vi "Process.vi"(8 "error in (no error)":errorcluster, 11 "SMO.UI.Example":refnum<class "SMO.UI.Example.lvclass">) -> (0 "error out":errorcluster, 3 "SMO.UI.Example out":refnum<class "SMO.UI.Example.lvclass">)   [LabVIEW 2013, in "SMO.UI.Example.lvclass"]
uses:
  SMO.UI.Example.lvclass
  SMO/Typedefs/Parent Call--Enum.ctl
  SMO.UI.Example.lvclass/SMO.UI.Example.ctl
  SMO.UI/SMO.UI.lvclass
  <vilib>/Utility/miscctls.llb/LVPointTypeDef.ctl
  SMO/Protected/ListThisLevelDependencies.vi
  SMO/reuse/CastArrayDependenciesToClusterOrClass.vi
  SMO.Example/SMO.Example.lvclass
  SMO/SMO.lvclass
panel:
  in  "------------ User Events -------":bool=TRUE
  out "Waveform Chart":cluster{"Flow 2":dbl, "Flow 1":dbl}(graph)
  out "Sensor 1 (LPM)":u8
  out "Sensor 2 (LPM)":u8
  in  "Valve":bool
  in  "Pump":bool
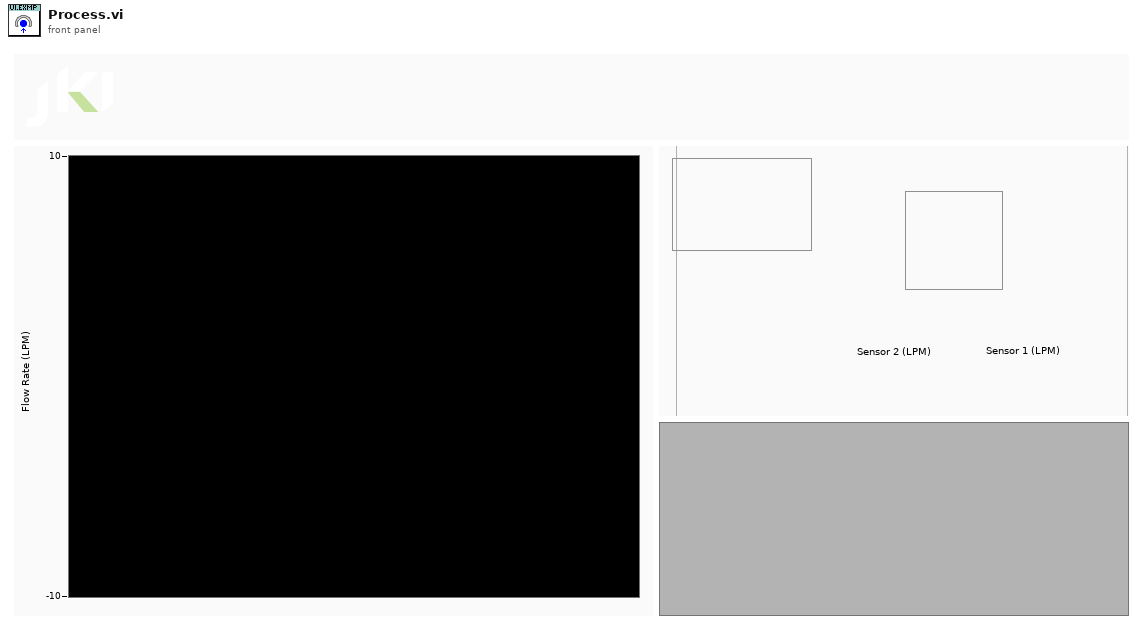
[diagram p1: front panel]
types:
  T1 = typedef "SMO.lvclass/Parent Call--Enum.ctl" = enum16{"Allows parent to run", "Does not request parent to run"}
  T2 = enum32{"invalid app kind", "Development System", "Run Time System", "Student Edition", "Embedded LabVIEW", "Evaluation", "Custom"}
  T3 = typedef "LVPointTypeDef.ctl" = cluster{"Horizontal":i16, "Vertical":i16}
  T4 = enum32{"Invalid", "Standard", "Closed", "Hidden", "Minimized", "Maximized"}
  T5 = typedef "SMO.UI.Example.lvclass/Dependencies--Cluster.ctl" = cluster{"SMO.Example":refnum<class "SMO.Example.lvclass">}
  T6 = cluster{"Core":cluster{"Current VI Reference":refnum<vi>, "Close Panel on Exit?":bool, "error":errorcluster}, "Self Ref":refnum<class "SMO.UI.Example.lvclass">, "Dependencies":T5, "Flow 1":dbl, "Flow 2":dbl}
  T7 = cluster{"Current VI Reference":refnum<vi>, "Close Panel on Exit?":bool, "error":errorcluster}
  T8 = typedef "SMO.lvclass/Protected Events.ctl" = cluster{"StopProcesses":refnum<user-event>, "AbortProcesses":refnum<user-event>, "Config Changed":refnum<user-event>}
  T9 = cluster{"Event Registration Refnum":refnum<event-registration>, "SMO.Example Public Events":refnum<event-registration>}
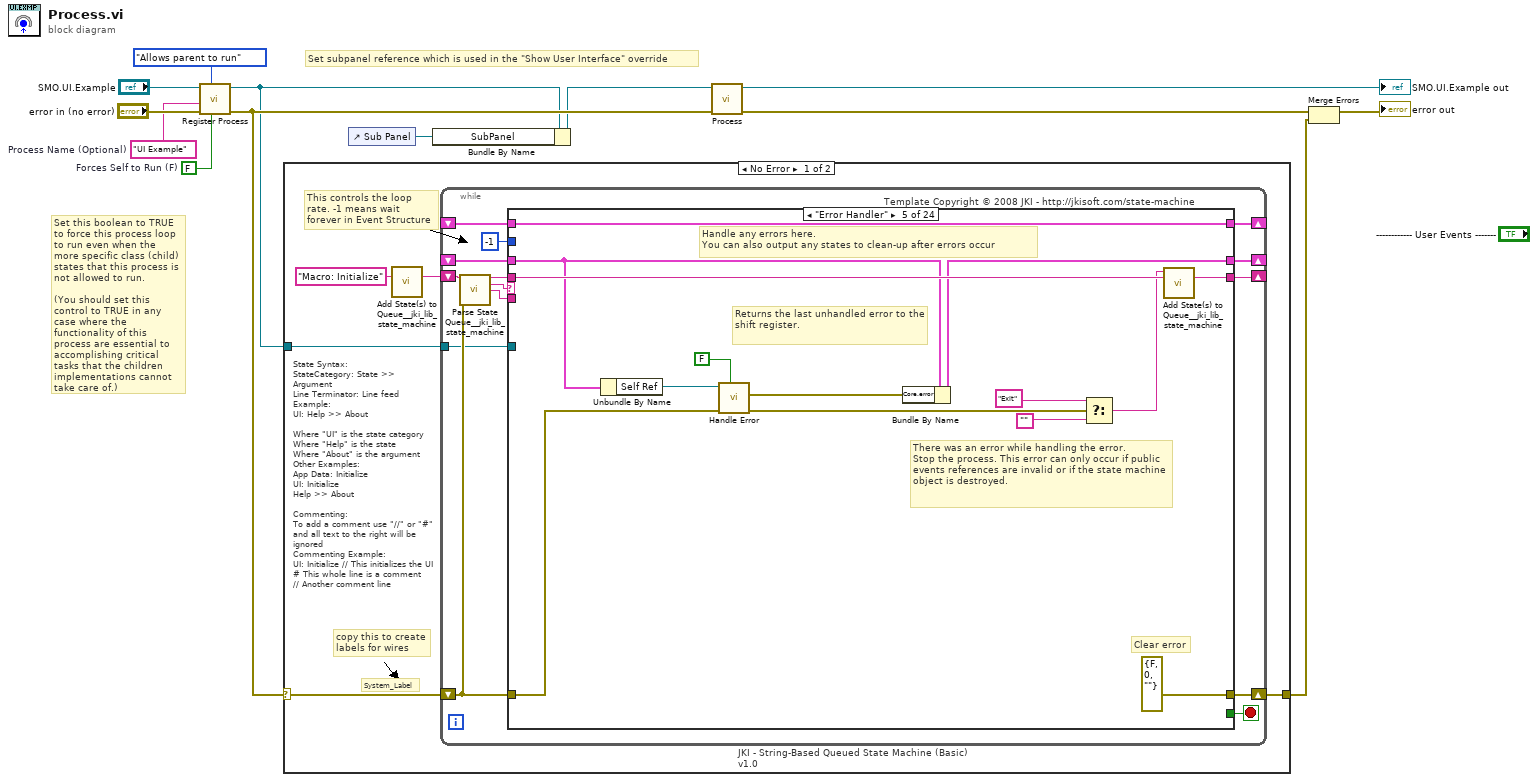
[diagram p0: block diagram]
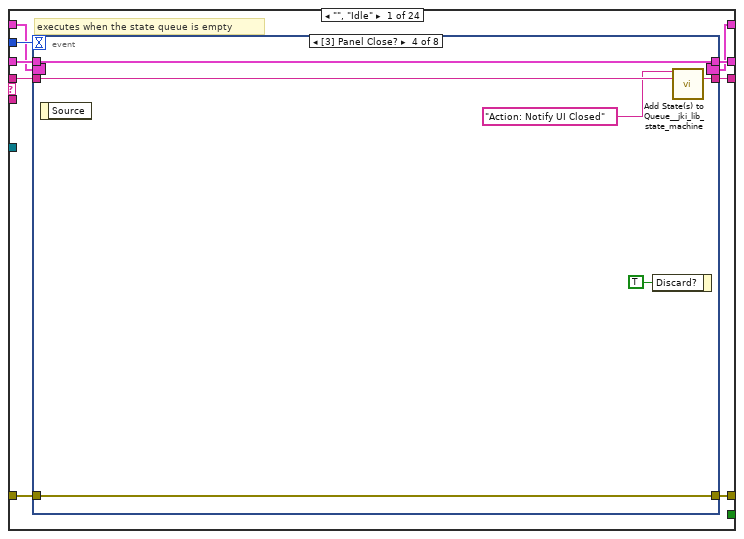
[diagram p2: hidden frame]
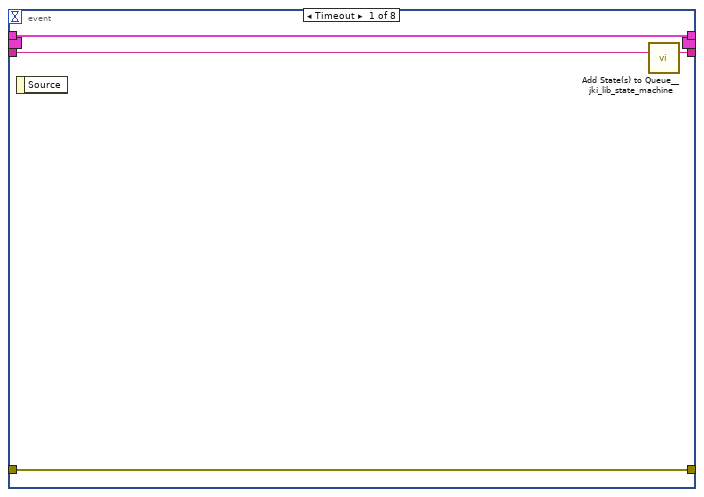
[diagram p3: hidden frame]
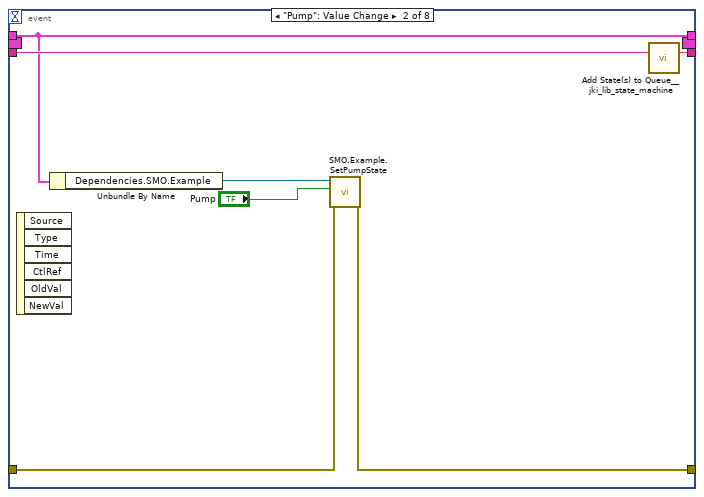
[diagram p4: hidden frame]
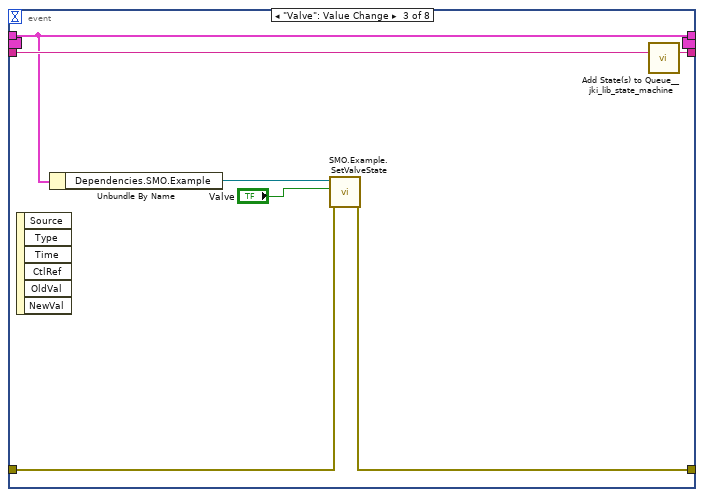
[diagram p5: hidden frame]
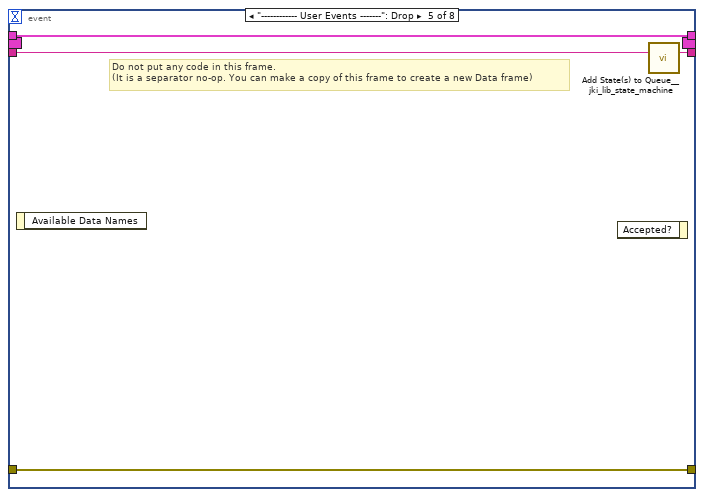
[diagram p6: hidden frame]
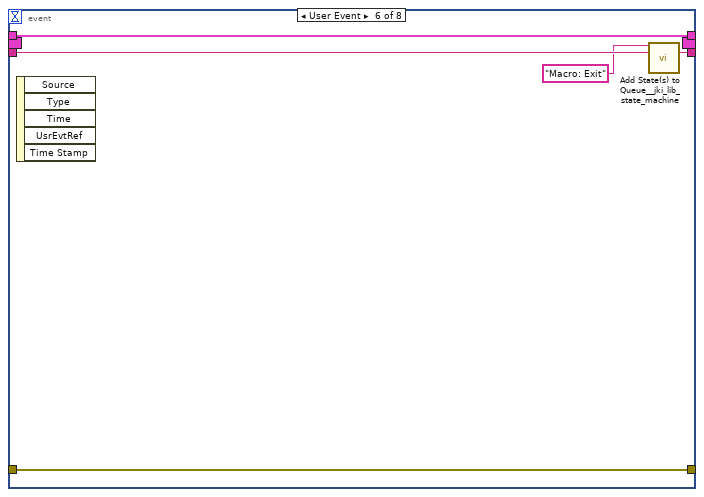
[diagram p7: hidden frame]
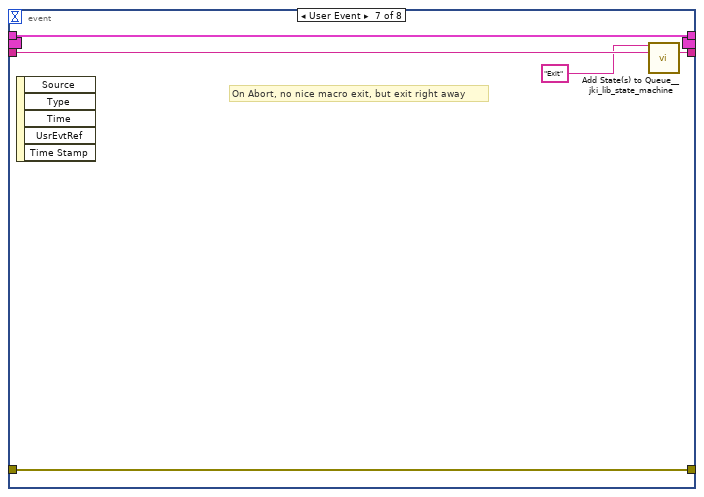
[diagram p8: hidden frame]
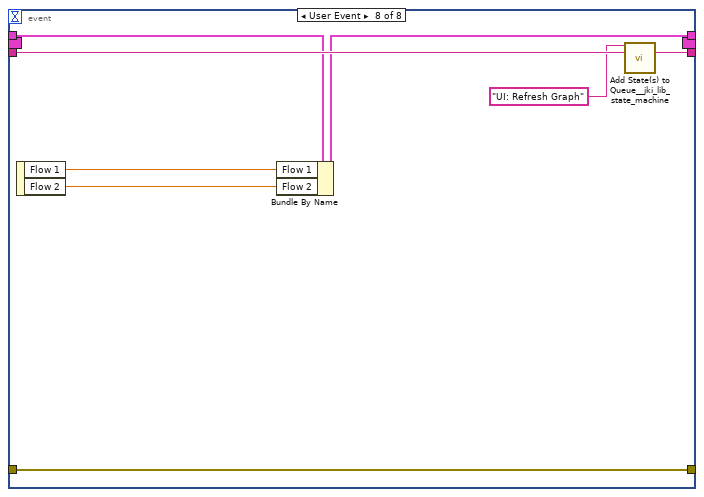
[diagram p9: hidden frame]
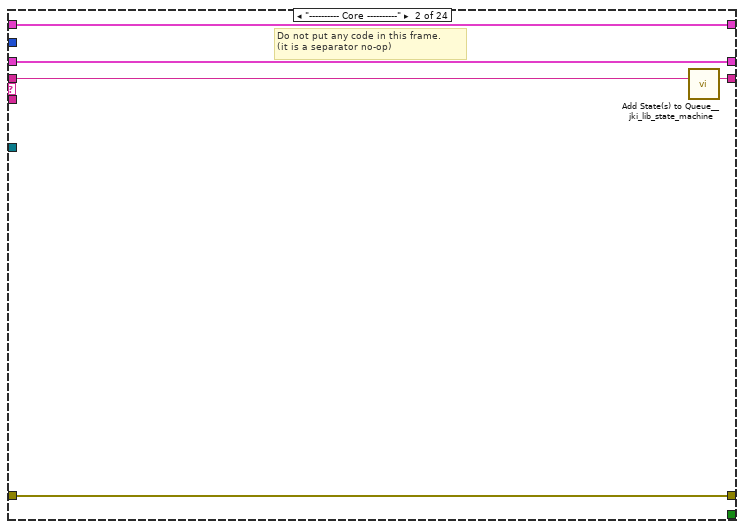
[diagram p10: hidden frame]
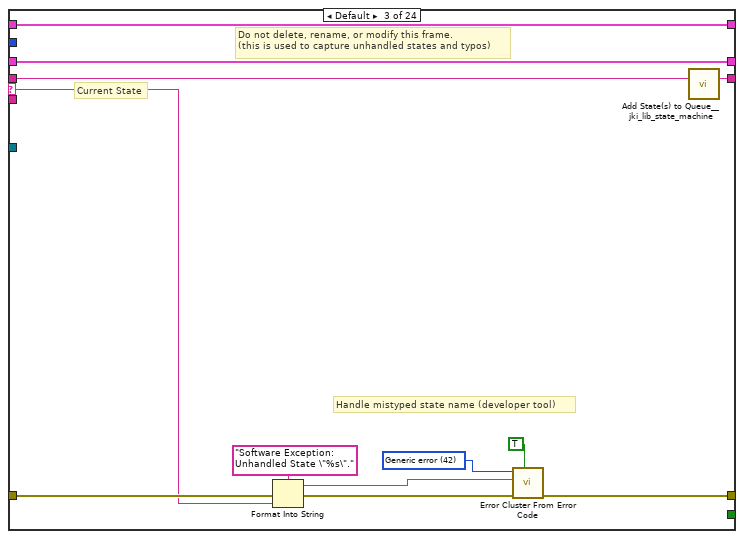
[diagram p11: hidden frame]
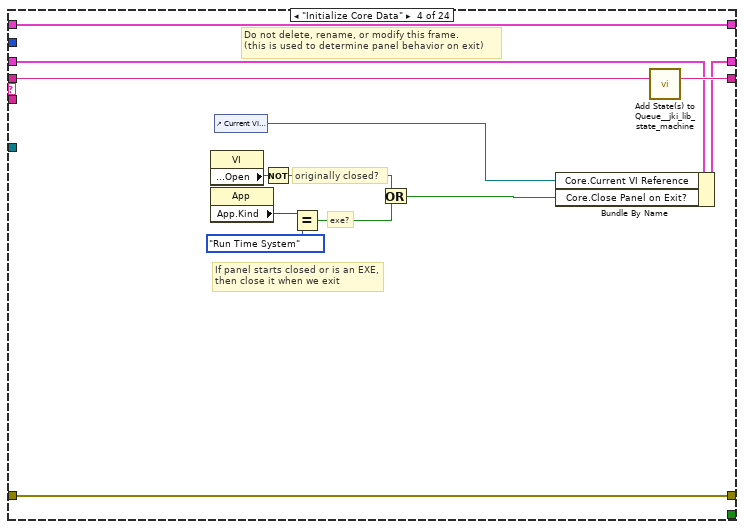
[diagram p12: hidden frame]
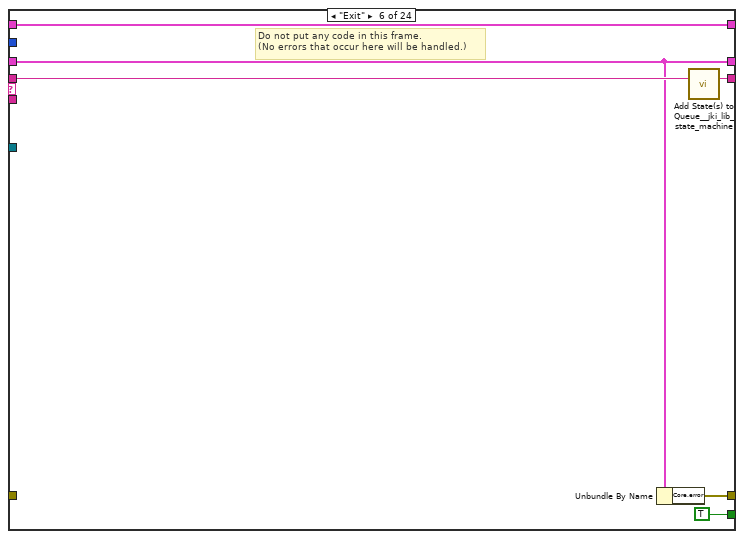
[diagram p13: hidden frame]
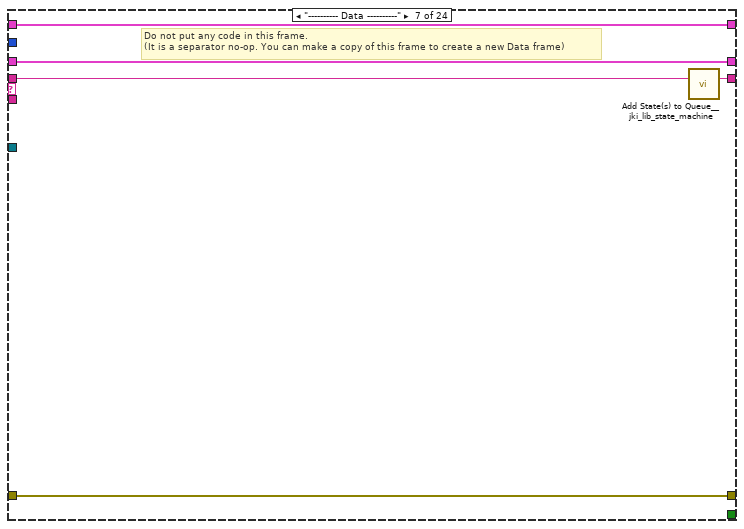
[diagram p14: hidden frame]
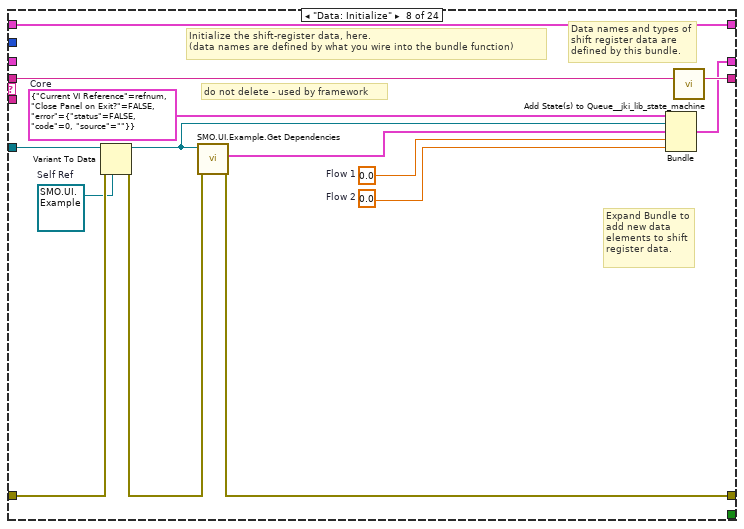
[diagram p15: hidden frame]
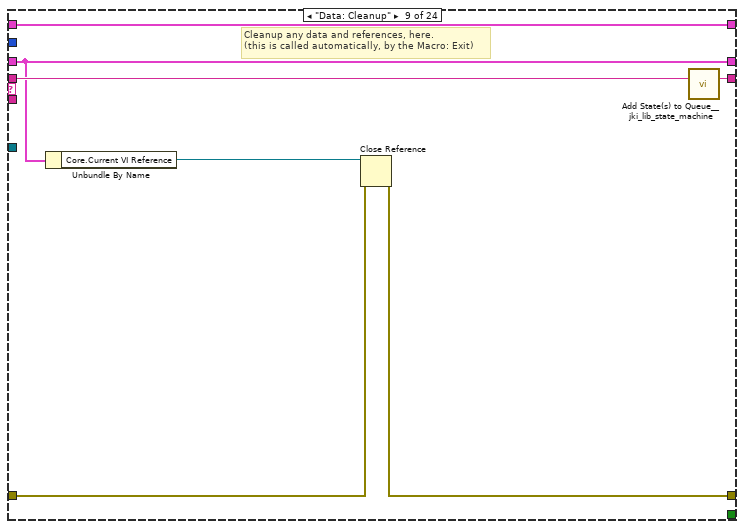
[diagram p16: hidden frame]
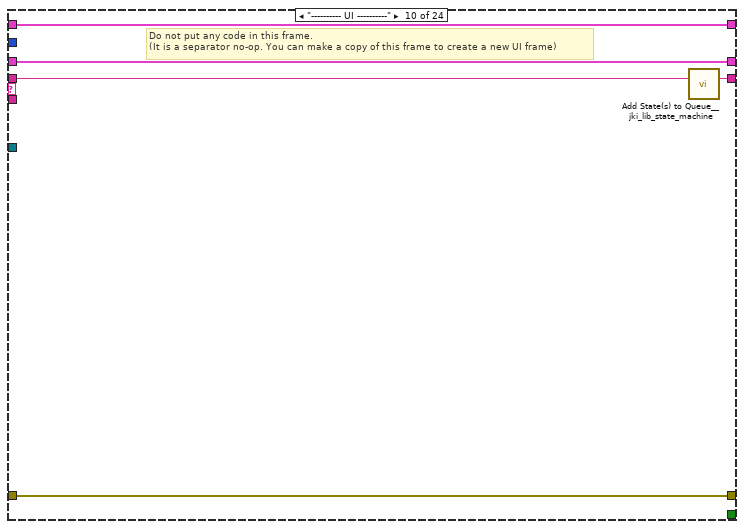
[diagram p17: hidden frame]
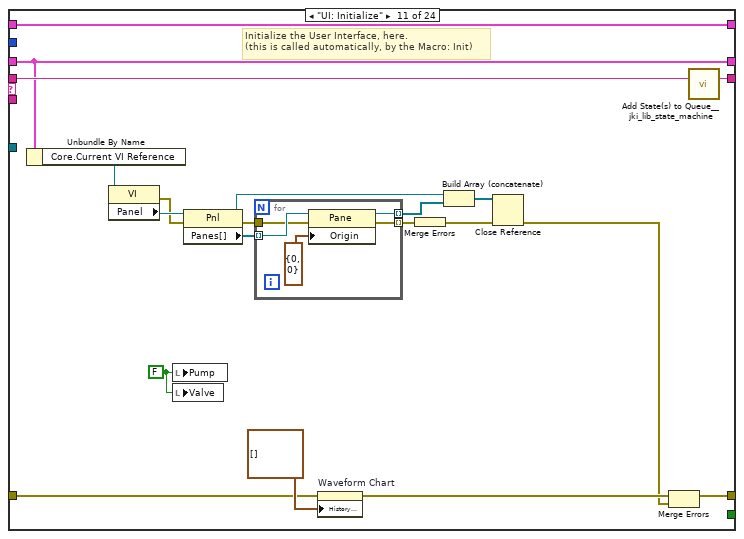
[diagram p18: hidden frame]
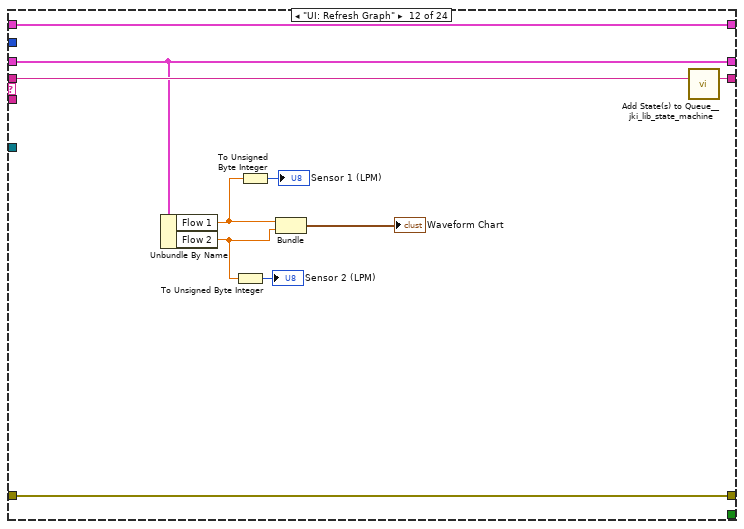
[diagram p19: hidden frame]
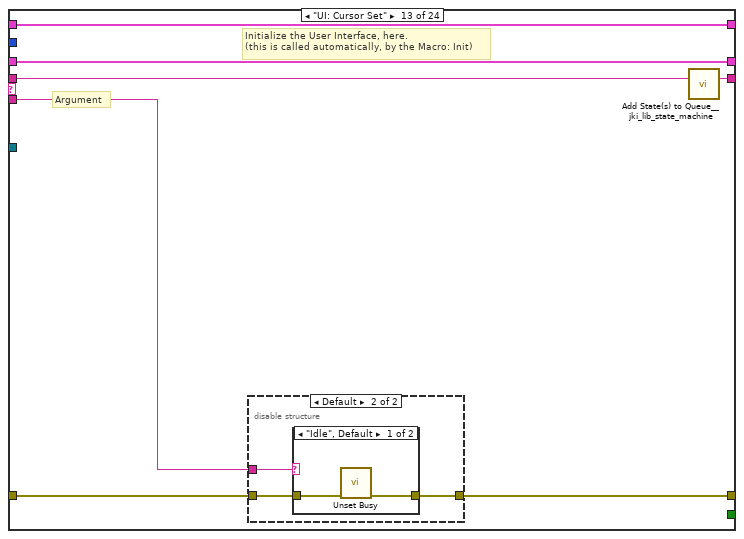
[diagram p20: hidden frame]
diagram:
  w1 = FALSE  # Forces Self to Run (F)
  w6 = "UI Example"  # Process Name (Optional)
  # "Set this boolean to TRUE to force this process loop to run even when the more specific class (child) states that this process is not allowed to run.\n\n(You should set this control to TRUE in any case where the functionality of this process are essential to accomplishing critical tasks that the children implementations cannot take care of.)"
  # "Set subpanel reference which is used in the \"Show User Interface\" override"
  n1 = call "Register Process.vi"("Forces Self to Run (F)"=w1, "Parent Call"=Parent_Call--Enum."Allows parent to run", "error in (no error)"="error in (no error)", "Process Name (optional)"=w6, "SMO"="SMO.UI.Example") -> ("error out"=w13:errorcluster, "SMO out"=w4:refnum<class "SMO.UI.Example.lvclass">)  [unwired: 5 in]
  n2 = case shown="No Error" w13 {
    selector: w13 -> [w15 w336]
    tunnel: w4 -> [w16 _]
    tunnel: [w14 w336] -> w11
    frame No Error {
      # "State Syntax:\nStateCategory: State >> Argument\nLine Terminator: Line feed\nExample:\nUI: Help >> About\n\nWhere \"UI\" is the state category\nWhere \"Help\" is the state\nWhere \"About\" is the argument\nOther Examples:\nApp Data: Initialize\nUI: Initialize\nHelp >> About\n\nCommenting:\nTo add a comment use \"//\" or \"#\" and all text to the right will be ignored\nCommenting Example:\nUI: Initialize // This initializes the UI\n# This whole line is a comment\n// Another comment line"
      # "copy this to create labels for wires"
      # "This controls the loop rate. -1 means wait forever in Event Structure"
      # "System_Label"
      n3 = call <vilib>:"Add State(s) to Queue__jki_lib_state_machine.vi"("State(s) in (\"\")"="Macro: Initialize") -> ("States Out"=w18:string)  [unwired: 14 in]
      n4 = while "JKI - String-Based Queued State Machine (Basic) v1.0" {
        shift-right: [w25] -> _
        shift-left: _ -> [w24]
        shift-right: [w28] -> w14
        shift-left: w15 -> [w22]
        shift-right: [w27] -> _
        shift-left: w18 -> [w29]
        tunnel: w16 -> [w21]
        shift-right: [w20] -> _
        shift-left: _ -> [w19]
        stop <- w26 stop-if-true
        # "Template Copyright © 2008 JKI - http://jkisoft.com/state-machine"
        n5 = call <vilib>:"Parse State Queue__jki_lib_state_machine.vi"("State Queue"=w29, "Error In (no error)"=w22) -> ("Remaining States"=w31:string, "Current State"=w32:string, "Arguments"=w30:string)  [unwired: 11 in]
        n6 = case shown="\"Error Handler\"" w32 {
          selector: w32 -> [_ _ w94 _ _ _ _ _ _ _ _ _ _ _ _ _ _ _ _ _ _ _ _ _]
          tunnel: w31 -> [w41 w92 w98 w117 w131 w137 w142 w156 w163 w168 w188 w203 w210 w226 w258 w267 w281 w286 w297 w302 w317 w323 w328 w335]
          tunnel: w30 -> [_ _ _ _ _ _ _ _ _ _ _ _ w204 w222 _ _ _ _ _ _ _ _ _ _]
          tunnel: w24 -> [w39 w89 w96 w108 w120 w133 w139 _ w158 w165 w183 w195 w208 w224 w255 w263 w272 w283 w294 w299 w315 w321 w325 w331]
          tunnel: [w38 w90 w100 w114 errorcluster {"status"=FALSE, "code"=0, "source"=""} ("error out") w132 w140 w145 w159 w166 w174 w194 w205 w219 w256 w265 w279 w284 w288 w300 w307 w319 w326 w329] -> w28
          tunnel: w22 -> [w37 w90 w99 w114 w122 _ w140 w153 w160 w166 w177 w194 w206 w220 w256 w265 w279 w284 w289 w300 w308 w319 w326 w330]
          tunnel: [w40 w91 w97 w116 w130 w136 w141 w155 w162 w167 w187 w202 w209 w225 w257 w266 w280 w285 w296 w301 w316 w322 w327 w334] -> w27
          tunnel: [_ _ _ _ _ TRUE _ _ _ _ _ _ _ _ _ _ _ _ _ _ _ _ _ _] -> w26
          tunnel: [w36 w89 w96 w115 w119 w133 w139 w154 w158 w165 w183 w195 w208 w224 w255 w263 w272 w283 w294 w299 w315 w321 w325 w331] -> w25
          tunnel: -1 ("Timeout") -> [w35 _ _ _ _ _ _ _ _ _ _ _ _ _ _ _ _ _ _ _ _ _ _ _]
          tunnel: w21 -> [_ _ _ _ _ _ _ w152 _ _ _ _ _ _ _ _ _ _ _ _ _ _ _ _]
          tunnel: [w33 w88 w93 w105 w128 w134 w138 w151 w157 w164 w184 w201 w207 w223 w254 w264 w273 w282 w295 w298 w310 w320 w324 w333] -> w20
          tunnel: w19 -> [w34 w88 w93 w105 w128 w134 w138 w151 w157 w164 w184 w201 w207 w223 w254 w264 w273 w282 w295 w298 _ w320 w324 w333]
          frame "", "Idle" {
            # "executes when the state queue is empty"
            n7 = event shown="[3] Panel Close?" {
              selector: w34 -> [_ _ _ _ _ _ _ _]
              dyn-events: [_ _ _ _ _ _ _ _] -> w33
              timeout: w35 -> [_ _ _ _ _ _ _ _]
              tunnel: w41 -> [w45 w52 w59 w65 w69 w74 w79 w87]
              tunnel: [w44 w51 w58 w64 w68 w73 w78 w86] -> w40
              tunnel: w39 -> [w42 w50 w57 w63 w66 w71 w76 w83]
              tunnel: [w43 w46 w54 w61 w67 w72 w77 w85] -> w38
              tunnel: w37 -> [w43 w47 w55 w61 w67 w72 w77 w85]
              tunnel: [w42 w50 w57 w63 w66 w71 w76 w84] -> w36
              event Timeout {
                n8 = event-data() -> ()  [unwired: 1 in, 1 out]
                n9 = call <vilib>:"Add State(s) to Queue__jki_lib_state_machine.vi"("State(s) in (\"\")"=w45) -> ("States Out"=w44:string)  [unwired: 14 in]
              }
              event "Pump": Value Change {
                n10 = event-data() -> ()  [unwired: 1 in, 6 out]
                n11 = Unbundle By Name(w50) -> ("Dependencies.SMO.Example"=w49:refnum<class "SMO.Example.lvclass">)
                n12 = call "SMO.Example.SetPumpState.vi"("error in (no error)"=w47, "Pump State"="Pump", "SMO.Example"=w49) -> ("error out"=w46:errorcluster)  [unwired: 7 in, 1 out]
                n13 = call <vilib>:"Add State(s) to Queue__jki_lib_state_machine.vi"("State(s) in (\"\")"=w52) -> ("States Out"=w51:string)  [unwired: 14 in]
              }
              event "Valve": Value Change {
                n14 = event-data() -> ()  [unwired: 1 in, 6 out]
                n15 = Unbundle By Name(w57) -> ("Dependencies.SMO.Example"=w56:refnum<class "SMO.Example.lvclass">)
                n16 = call "SMO.Example.SetValveState.vi"("error in (no error)"=w55, "Valve State"="Valve", "SMO.Example"=w56) -> ("error out"=w54:errorcluster)  [unwired: 7 in, 1 out]
                n17 = call <vilib>:"Add State(s) to Queue__jki_lib_state_machine.vi"("State(s) in (\"\")"=w59) -> ("States Out"=w58:string)  [unwired: 14 in]
              }
              event Panel Close? {
                n18 = event-data() -> ()  [unwired: 1 in, 1 out]
                n19 = event-data("Discard?"=TRUE) -> ()  [unwired: 1 in, 1 out]
                n20 = call <vilib>:"Add State(s) to Queue__jki_lib_state_machine.vi"("State(s) in Front (\"\")"="Action: Notify UI Closed" ("State(s) in Front (\"\")"), "State(s) in (\"\")"=w65) -> ("States Out"=w64:string)  [unwired: 13 in]
              }
              event "------------ User Events -------": Drop {
                # "Do not put any code in this frame.\n(It is a separator no-op. You can make a copy of this frame to create a new Data frame)"
                n21 = event-data() -> ()  [unwired: 1 in, 1 out]
                n22 = event-data() -> ()  [unwired: 2 in, 1 out]
                n23 = call <vilib>:"Add State(s) to Queue__jki_lib_state_machine.vi"("State(s) in (\"\")"=w69) -> ("States Out"=w68:string)  [unwired: 14 in]
              }
              event User Event {
                n24 = event-data() -> ()  [unwired: 1 in, 5 out]
                n25 = call <vilib>:"Add State(s) to Queue__jki_lib_state_machine.vi"("State(s) in Front (\"\")"="Macro: Exit", "State(s) in (\"\")"=w74) -> ("States Out"=w73:string)  [unwired: 13 in]
              }
              event User Event {
                # "On Abort, no nice macro exit, but exit right away"
                n26 = event-data() -> ()  [unwired: 1 in, 5 out]
                n27 = call <vilib>:"Add State(s) to Queue__jki_lib_state_machine.vi"("State(s) in Front (\"\")"="Exit", "State(s) in (\"\")"=w79) -> ("States Out"=w78:string)  [unwired: 13 in]
              }
              event User Event {
                n28 = event-data() -> ("Flow 1"=w82:dbl, "Flow 2"=w81:dbl)  [unwired: 1 in]
                n29 = Bundle By Name(cluster=w83, "Flow 1"=w82, "Flow 2"=w81) -> (w84:T6)
                n30 = call <vilib>:"Add State(s) to Queue__jki_lib_state_machine.vi"("State(s) in Front (\"\")"="UI: Refresh Graph", "State(s) in (\"\")"=w87) -> ("States Out"=w86:string)  [unwired: 13 in]
              }
            }
          }
          frame "---------- Core ----------" {
            # "Do not put any code in this frame.\n(it is a separator no-op)"
            n31 = call <vilib>:"Add State(s) to Queue__jki_lib_state_machine.vi"("State(s) in (\"\")"=w92) -> ("States Out"=w91:string)  [unwired: 14 in]
          }
          frame Default {
            w103 = 42 items=["No error", "Argument error", "Memory is full", "Out of zone", "End of file", "File already open", "Generic file I/O error", "File not found", "File permission error", "Disk is full", "Duplicate path", "Too many files open", "System feature not enabled", "Resource file not found", "Cannot add resource", "Resource not found", "Image not found", "Image memory error", "Pen does not exist", "Config type invalid", "Config token not found", "Config parse error", "Config memory error", "Bad external code format", "Bad external code offset", "External code not present", "Null window", "Destroy window error", "Null menu", "Print aborted", "Bad print record", "Print driver error", "Windows error during printing", "Memory error during printing", "Print dialog error", "Generic print error", "Invalid device refnum", "Device not found", "Device parameter error", "Device unit error", "Cannot open device", "Device call aborted", "Generic error", "Cancelled by user", "Object ID too low", "Object ID too high", "Object not in heap", "Unknown heap", "Unknown object (invalid DefProc)", "Unknown object (DefProc not in table)", "Message out of range", "Invalid (null) method", "Unknown message", "Manager call not supported", "Bad address", "Network operation in progress", "Network operation timed out", "Connection is busy", "Network attribute not supported", "Network error", "Address in use", "System out of memory", "Connection aborted", "Connection refused", "Not connected", "Already connected", "Connection closed", "Initialization error (interapplication manager)", "Bad occurrence", "Wait on unbound occurrence handler", "Occurrence queue overflow", "Datalog type conflict", "Unused", "Unrecognized type (interapplication manager)", "Memory corrupt", "Failed to make temporary DLL", "Old CIN version", "Drag socket not found", "Failed to load drop-object", "Failed to register OLE object", "Failed to release OLE object", "Format specifier type mismatch", "Unknown format specifier", "Too few format specifiers", "Too many format specifiers", "Scan failed", "Newer CIN version", "Error converting to variant", "Runtime menu error", "Password tampered", "Variant attribute not found", "Incompatible variant data type", "Event data is not available", "Event Store is not present", "Occurrence is not found", "Event Queue is not created", "Event info is not available", "Refnum passed is NULL", "Error retrieving Class GUID", "Error retrieving CoClass GUID", "Error retrieving TypeLib GUID.", "Bad built application magic bytes.", "Specific driver is different from the specific driver associated with the Logical Name.", "There is no session opened to the class driver.", "Max Error", "MAX - Error with config objects", "MAX - Error loading configuration", "MAX - Group not supported"]
            # "Current State"
            # "Do not delete, rename, or modify this frame.\n(this is used to capture unhandled states and typos)"
            # "Handle mistyped state name (developer tool)"
            n32 = Format Into String(format string="Software Exception: Unhandled State \"%s\"." ("message"), error in=w99, w94) -> (resulting string=w102:string, error out=w101:errorcluster)  [unwired: 1 in]
            n33 = call <vilib>:"Error Cluster From Error Code.vi"("show call chain? (False)"=TRUE, "error in (no error)"=w101, "error message (\"\")"=w102, "error code (0)"=w103) -> ("error out"=w100:errorcluster)  [unwired: 5 in]
            n34 = call <vilib>:"Add State(s) to Queue__jki_lib_state_machine.vi"("State(s) in (\"\")"=w98) -> ("States Out"=w97:string)  [unwired: 14 in]
          }
          frame "Initialize Core Data" {
            # "Do not delete, rename, or modify this frame.\n(this is used to determine panel behavior on exit)"
            # "originally closed?"
            # "exe?"
            # "If panel starts closed or is an EXE, then close it when we exit"
            n35 = property class="VI"() -> ("Front Panel.Open"=w113:bool)  [unwired: 2 in, 2 out]
            n36 = property class="App"() -> ("App.Kind"=w112:T2)  [unwired: 2 in, 2 out]
            n37 = control-ref of="Current VI Reference"() -> (w106:refnum<vi>)
            n38 = Not(x=w113) -> (.not. x?=w110:bool)
            n39 = Equal?(x=w112, y=T2."Run Time System" ("Application:Kind")) -> (x = y?=w109:bool)
            n40 = Or(x=w110, y=w109) -> (x .or. y?=w107:bool)
            n41 = Bundle By Name(cluster=w108, "Core.Current VI Reference"=w106, "Core.Close Panel on Exit?"=w107) -> (w115:T6)
            n42 = call <vilib>:"Add State(s) to Queue__jki_lib_state_machine.vi"("State(s) in (\"\")"=w117) -> ("States Out"=w116:string)  [unwired: 14 in]
          }
          frame "Error Handler" {
            # "Returns the last unhandled error to the shift register."
            # "There was an error while handling the error.\nStop the process. This error can only occur if public events references are invalid or if the state machine object is destroyed."
            # "Handle any errors here.\nYou can also output any states to clean-up after errors occur"
            # "Clear error"
            n43 = Unbundle By Name(w120) -> ("Self Ref"=w127:refnum<class "SMO.UI.Example.lvclass">)
            n44 = call-dynamic "Handle Error.vi"("Stop on Unhandled Error (T)"=FALSE, "error in"=w122, "SMO"=w127) -> ("handling error"=w125:errorcluster, "Unhandled error"=w126:errorcluster)  [unwired: 6 in, 1 out]
            n45 = Bundle By Name(cluster=w120, "Core.error"=w126) -> (w119:T6)
            n46 = Select(t="Exit", s=w125, f="") -> (s? t:f=w121:string)
            n47 = call <vilib>:"Add State(s) to Queue__jki_lib_state_machine.vi"("State(s) in Front (\"\")"=w121, "State(s) in (\"\")"=w131) -> ("States Out"=w130:string)  [unwired: 13 in]
          }
          frame "Exit" {
            # "Do not put any code in this frame.\n(No errors that occur here will be handled.)"
            n48 = Unbundle By Name(w133) -> ("Core.error"=w132:errorcluster)
            n49 = call <vilib>:"Add State(s) to Queue__jki_lib_state_machine.vi"("State(s) in (\"\")"=w137) -> ("States Out"=w136:string)  [unwired: 14 in]
          }
          frame "---------- Data ----------" {
            # "Do not put any code in this frame.\n(It is a separator no-op. You can make a copy of this frame to create a new Data frame)"
            n50 = call <vilib>:"Add State(s) to Queue__jki_lib_state_machine.vi"("State(s) in (\"\")"=w142) -> ("States Out"=w141:string)  [unwired: 14 in]
          }
          frame "Data: Initialize" {
            w144 = 0.0  # Flow 1
            w143 = 0.0  # Flow 2
            w149 = refnum<class "SMO.UI.Example.lvclass"> refnum  # Self Ref
            w150 = T7 {"Current VI Reference"=refnum, "Close Panel on Exit?"=FALSE, "error"={"status"=FALSE, "code"=0, "source"=""}}  # Core
            # "do not delete - used by framework"
            # "Expand Bundle to add new data elements to shift register data."
            # "Data names and types of shift register data are defined by this bundle."
            # "Initialize the shift-register data, here.\n(data names are defined by what you wire into the bundle function)"
            n51 = Variant To Data(error in=w153, type=w149, Variant=w152) -> (data=w147:refnum<class "SMO.UI.Example.lvclass">, error out=w146:errorcluster)
            n52 = call "SMO.UI.Example.Get Dependencies.vi"("error in (no error)"=w146, "SMO UI.Template in"=w147) -> ("error out"=w145:errorcluster, "Dependencies"=w148:T5)  [unwired: 7 in, 1 out]
            n53 = Bundle("Core"=w150, "Self Ref"=w147, "Dependencies"=w148, "Flow 1"=w144, "Flow 2"=w143) -> (w154:T6)  [unwired: 1 in]
            n54 = call <vilib>:"Add State(s) to Queue__jki_lib_state_machine.vi"("State(s) in (\"\")"=w156) -> ("States Out"=w155:string)  [unwired: 14 in]
          }
          frame "Data: Cleanup" {
            # "Cleanup any data and references, here.\n(this is called automatically, by the Macro: Exit)"
            n55 = Unbundle By Name(w158) -> ("Core.Current VI Reference"=w161:refnum<vi>)
            n56 = Close Reference(reference=w161, error in (no error)=w160) -> (error out=w159:errorcluster)
            n57 = call <vilib>:"Add State(s) to Queue__jki_lib_state_machine.vi"("State(s) in (\"\")"=w163) -> ("States Out"=w162:string)  [unwired: 14 in]
          }
          frame "---------- UI ----------" {
            # "Do not put any code in this frame.\n(It is a separator no-op. You can make a copy of this frame to create a new UI frame)"
            n58 = call <vilib>:"Add State(s) to Queue__jki_lib_state_machine.vi"("State(s) in (\"\")"=w168) -> ("States Out"=w167:string)  [unwired: 14 in]
          }
          frame "UI: Initialize" {
            w186 = FALSE ("Pump")
            # "Initialize the User Interface, here.\n(this is called automatically, by the Macro: Init)"
            n59 = Unbundle By Name(w183) -> ("Core.Current VI Reference"=w182:refnum<vi>)
            n60 = property class="VI"(reference=w182) -> (error out=w179:errorcluster, "Panel"=w181:refnum<vi>)  [unwired: 1 in, 1 out]
            n61 = local write "Pump"(w186) -> ()
            n62 = local write "Valve"(w186) -> ()
            n63 = property class="Pnl"(reference=w181, error in=w179) -> (reference out=w173:refnum<vi>, error out=w178:errorcluster, "Panes[]"=w180:refnum<vi>[])
            n64 = for {
              tunnel: w180 -> [w193] mode=indexing
              tunnel: w178 -> [w191]
              tunnel: [w190] -> w176 mode=indexing
              tunnel: [w189] -> w172 mode=indexing
              n65 = property class="Pane"(reference=w193, error in=w191, "Origin"=T3 {"Horizontal"=0, "Vertical"=0}) -> (reference out=w189:refnum<vi>, error out=w190:errorcluster)
            }
            n66 = property on="Waveform Chart" class="WFChart (strict)"(error in=w177, "History Data"=cluster{"Flow 2":dbl, "Flow 1":dbl}[] []) -> (error out=w175:errorcluster)  [unwired: 1 in, 1 out]
            n67 = Merge Errors(w176) -> (w171:errorcluster)
            n68 = Build Array (concatenate)(w173, w172) -> (w169:refnum<vi>[])
            n69 = Close Reference(reference=w169, error in (no error)=w171) -> (error out=w170:errorcluster)
            n70 = Merge Errors(w175, w170) -> (w174:errorcluster)
            n71 = call <vilib>:"Add State(s) to Queue__jki_lib_state_machine.vi"("State(s) in (\"\")"=w188) -> ("States Out"=w187:string)  [unwired: 14 in]
          }
          frame "UI: Refresh Graph" {
            n72 = Unbundle By Name(w195) -> ("Flow 1"=w198:dbl, "Flow 2"=w199:dbl)
            n73 = To Unsigned Byte Integer(number=w199) -> (unsigned 8bit integer=→"Sensor 2 (LPM)":u8)
            n74 = To Unsigned Byte Integer(number=w198) -> (unsigned 8bit integer=→"Sensor 1 (LPM)":u8)
            n75 = Bundle("Flow 1"=w198, "Flow 2"=w199) -> (→"Waveform Chart":cluster{"Flow 1":dbl, "Flow 2":dbl})  [unwired: 1 in]
            n76 = call <vilib>:"Add State(s) to Queue__jki_lib_state_machine.vi"("State(s) in (\"\")"=w203) -> ("States Out"=w202:string)  [unwired: 14 in]
          }
          frame "UI: Cursor Set" {
            # "Argument"
            # "Initialize the User Interface, here.\n(this is called automatically, by the Macro: Init)"
            n77 = disable-structure shown="Default" {
              disable-tunnel: w206 -> [w211 w214]
              disable-tunnel: [w211 w213] -> w205
              disable-tunnel: w204 -> [_ w212]
              frame condition #0 {
              }
              frame condition #1 (active) {
                n78 = case shown="\"Idle\", Default" w212 {
                  tunnel: w214 -> [w216 w218]
                  tunnel: [w215 w217] -> w213
                  frame "Idle", Default {
                    n79 = call <vilib>:"Unset Busy.vi"("error in (no error)"=w216) -> ("error out"=w215:errorcluster)  [unwired: 10 in]
                  }
                  frame "Busy" {
                    n80 = call <vilib>:"Set Busy.vi"("error in (no error)"=w218) -> ("error out"=w217:errorcluster)  [unwired: 9 in, 1 out]
                  }
                }
              }
            }
            n81 = call <vilib>:"Add State(s) to Queue__jki_lib_state_machine.vi"("State(s) in (\"\")"=w210) -> ("States Out"=w209:string)  [unwired: 14 in]
          }
          frame "UI: Front Panel State" {
            # "Argument"
            # "Set Front Panel Open or Closed\n(Usage: \"UI: Front Panel State >> Open|Close\")"
            n82 = Unbundle By Name(w224) -> ("Core.Current VI Reference"=w221:refnum<vi>)
            n83 = disable-structure shown="Default" {
              disable-tunnel: w220 -> [w230 w253]
              disable-tunnel: [w229 w253] -> w219
              disable-tunnel: w221 -> [w228 _]
              disable-tunnel: w222 -> [w227 _]
              frame condition #0 (active) {
                n84 = case shown="\"Open\", Default" w227 {
                  tunnel: w230 -> [w234 w247]
                  tunnel: [w236 w248] -> w229
                  tunnel: w228 -> [w235 w245]
                  frame "Open", Default {
                    # "Open FP if not open or invalid"
                    n85 = property class="VI"(reference=w235, error in=w234) -> (reference out=w232:refnum<vi>, error out=w233:errorcluster, "FP.State"=w231:T4)
                    n86 = case shown="Default" w231 {
                      tunnel: [w239 w242] -> w236
                      tunnel: w233 -> [w238 w242]
                      tunnel: w232 -> [w237 _]
                      frame Default {
                        n87 = invoke class="VI" method="FP.Open"(reference=w237, error in=w238, "Activate"=TRUE, "State"=T4."Standard") -> (error out=w239:errorcluster)  [unwired: 1 in, 4 out]
                      }
                      frame "Invalid", "Standard" {
                      }
                    }
                  }
                  frame "Close" {
                    # "Close FP is not Closed or Invalid"
                    n88 = property class="VI"(reference=w245, error in=w247) -> (reference out=w244:refnum<vi>, error out=w246:errorcluster, "FP.State"=w243:T4)
                    n89 = case shown="Default" w243 {
                      tunnel: [w249 w252] -> w248
                      tunnel: w246 -> [w249 w251]
                      tunnel: w244 -> [_ w250]
                      frame "Invalid", "Closed" {
                      }
                      frame Default {
                        n90 = invoke class="VI" method="FP.Close"(reference=w250, error in=w251) -> (error out=w252:errorcluster)  [unwired: 1 in, 2 out]
                      }
                    }
                  }
                }
              }
              frame condition #1 {
              }
            }
            n91 = call <vilib>:"Add State(s) to Queue__jki_lib_state_machine.vi"("State(s) in (\"\")"=w226) -> ("States Out"=w225:string)  [unwired: 14 in]
          }
          frame "---------- Macro ----------" {
            # "Do not put any code in this frame.\n(It is a separator no-op. You can make a copy of this frame to create a new Macro frame)"
            n92 = call <vilib>:"Add State(s) to Queue__jki_lib_state_machine.vi"("State(s) in (\"\")"=w258) -> ("States Out"=w257:string)  [unwired: 14 in]
          }
          frame "Macro: Initialize" {
            w261 = "UI: Initialize\n//UI: Front Panel State >> Open"  # UI: Initialize //UI: Front Panel State >> Open
            # "Initialization Macro\n(This is called once, when the VI starts)"
            n93 = call <vilib>:"Add State(s) to Queue__jki_lib_state_machine.vi"("State(s) in Front (\"\")"="Data: Initialize\nInitialize Core Data\nEvents: Register", "State(s) in (\"\")"="Process: Sync", "State(s) at Back (\"\")"=w261) -> ("States Out"=w260:string)  [unwired: 12 in]
            n94 = call <vilib>:"Add State(s) to Queue__jki_lib_state_machine.vi"("State(s) in Front (\"\")"=w260, "State(s) in (\"\")"=w267) -> ("States Out"=w266:string)  [unwired: 13 in]
          }
          frame "Macro: Exit" {
            # "Exit Macro\n(This is called once, when the VI exits)"
            n95 = Unbundle By Name(w272) -> ("Core.Close Panel on Exit?"=w278:bool)
            n96 = Select(t="//UI: Front Panel State >> Close", s=w278, f="") -> (s? t:f=w275:string)
            n97 = call <vilib>:"Add State(s) to Queue__jki_lib_state_machine.vi"("State(s) in Front (\"\")"="Data: Cleanup\nEvents: Unregister", "State(s) in (\"\")"="Process: Sync", "State(s) at Back (\"\")"="Exit") -> ("States Out"=w269:string)  [unwired: 12 in]
            n98 = call <vilib>:"Add State(s) to Queue__jki_lib_state_machine.vi"("State(s) in (\"\")"=w275, "State(s) at Back (\"\")"=w269) -> ("States Out"=w274:string)  [unwired: 13 in]
            n99 = call <vilib>:"Add State(s) to Queue__jki_lib_state_machine.vi"("State(s) in Front (\"\")"=w274, "State(s) in (\"\")"=w281) -> ("States Out"=w280:string)  [unwired: 13 in]
          }
          frame "---------- Process ----------" {
            # "Template Separator\n(You can make a copy of, or modify, this frame)"
            n100 = call <vilib>:"Add State(s) to Queue__jki_lib_state_machine.vi"("State(s) in (\"\")"=w286) -> ("States Out"=w285:string)  [unwired: 14 in]
          }
          frame "Process: Sync" {
            n101 = Unbundle By Name(w294) -> ("Self Ref"=w290:refnum<class "SMO.UI.Example.lvclass">)
            n102 = call "WaitOnProcessSync.vi"("error in (no error)"=w289, "SMO"=w290) -> ("error out"=w288:errorcluster, "Don't run?"=w293:bool)  [unwired: 7 in, 1 out]
            n103 = Select(t="Data: Cleanup\nEvents: Unregister\nExit", s=w293, f="") -> (s? t:f=w287:string)
            n104 = call <vilib>:"Add State(s) to Queue__jki_lib_state_machine.vi"("State(s) in Front (\"\")"=w287, "State(s) in (\"\")"=w297) -> ("States Out"=w296:string)  [unwired: 13 in]
          }
          frame "---------- Events ----------" {
            # "Template Separator\n(You can make a copy of, or modify, this frame)"
            n105 = call <vilib>:"Add State(s) to Queue__jki_lib_state_machine.vi"("State(s) in (\"\")"=w302) -> ("States Out"=w301:string)  [unwired: 14 in]
          }
          frame "Events: Register" {
            # "Clear error when dependency not created. (Demo only)"
            # "Dependency Public Events"
            # "Base Class Protected Events"
            n106 = Unbundle By Name(w315) -> ("Self Ref"=w309:refnum<class "SMO.UI.Example.lvclass">)
            n107 = Unbundle By Name(w315) -> ("Dependencies.SMO.Example"=w313:refnum<class "SMO.Example.lvclass">)
            n108 = call "SMO.Example.GetPublicEventsRegistration.vi"("SMO.Example"=w313) -> ("error out"=w304:errorcluster, "SMO.Example Public Events"=w312:refnum<event-registration>)  [unwired: 8 in, 1 out]
            n109 = call <vilib>:"Clear Errors.vi"("error in (no error)"=w304) -> ("error out"=w303:errorcluster)  [unwired: 6 in]
            n110 = call "GetProtectedEvents.vi"("SMO"=w309) -> ("error out"=w305:errorcluster, "SMO Protected Events"=w314:T8)  [unwired: 8 in, 1 out]
            n111 = register-events(w314) -> (reference out=w311:refnum<event-registration>, error out=w306:errorcluster)  [unwired: 2 in]
            n112 = Merge Errors(w306, w305, w303, w308) -> (w307:errorcluster)
            n113 = Bundle("Event Registration Refnum"=w311, "SMO.Example Public Events"=w312) -> (w310:T9)  [unwired: 1 in]
            n114 = call <vilib>:"Add State(s) to Queue__jki_lib_state_machine.vi"("State(s) in (\"\")"=w317) -> ("States Out"=w316:string)  [unwired: 14 in]
          }
          frame "Events: Unregister" {
            n115 = Unregister For Events(event registration refnum=w320, error in=w319) -> (error out=w318:errorcluster)
            n116 = call <vilib>:"Clear Errors.vi"("error in (no error)"=w318) -> ()  [unwired: 6 in, 1 out]
            n117 = call <vilib>:"Add State(s) to Queue__jki_lib_state_machine.vi"("State(s) in (\"\")"=w323) -> ("States Out"=w322:string)  [unwired: 14 in]
          }
          frame "---------Action---------" {
            # "Action Separator\n(You can make a copy of, or modify, this frame)"
            n118 = call <vilib>:"Add State(s) to Queue__jki_lib_state_machine.vi"("State(s) in (\"\")"=w328) -> ("States Out"=w327:string)  [unwired: 14 in]
          }
          frame "Action: Notify UI Closed" {
            # "Notify that the UI has closed"
            # "Action Separator\n(You can make a copy of, or modify, this frame)"
            n119 = Unbundle By Name(w331) -> ("Self Ref"=w332:refnum<class "SMO.UI.Example.lvclass">)
            n120 = call "Hide.vi"("error in (no error)"=w330, "SMO.UI"=w332) -> ("error out"=w329:errorcluster)  [unwired: 8 in, 1 out]
            n121 = call <vilib>:"Add State(s) to Queue__jki_lib_state_machine.vi"("State(s) in (\"\")"=w335) -> ("States Out"=w334:string)  [unwired: 14 in]
          }
        }
      }
    }
    frame Error {
    }
  }
  n122 = control-ref of="Sub Panel"() -> (w2:refnum<vi>)
  n123 = Bundle By Name(cluster=w4, "SubPanel"=w2) -> (w3:refnum<class "SMO.UI.Example.lvclass">)
  n124 = call-parent "Process.vi"("error in (no error)"=w13, "SMO.UI"=w3) -> ("error out"=w12:errorcluster, "SMO.UI out"=→"SMO.UI.Example out":refnum<class "SMO.UI.Example.lvclass">)  [unwired: 8 in]
  n125 = Merge Errors(w12, w11) -> (→"error out":errorcluster)
